vi "open.vi"(8 "error in (no error)":errorcluster caption="错误输入（无错误）", 11 "TCP 输入":refnum<class "TCP.lvclass">) -> (0 "error out":errorcluster caption="错误输出", 3 "TCP 输出":refnum<class "TCP.lvclass">)   [LabVIEW 2016, in "中水三立SQL数据传输.lvlib" / "TCP.lvclass"]
uses:
  TCP.lvclass
  data_inter/data_inter.lvclass/data_inter.ctl
  data_inter/data_inter.lvclass
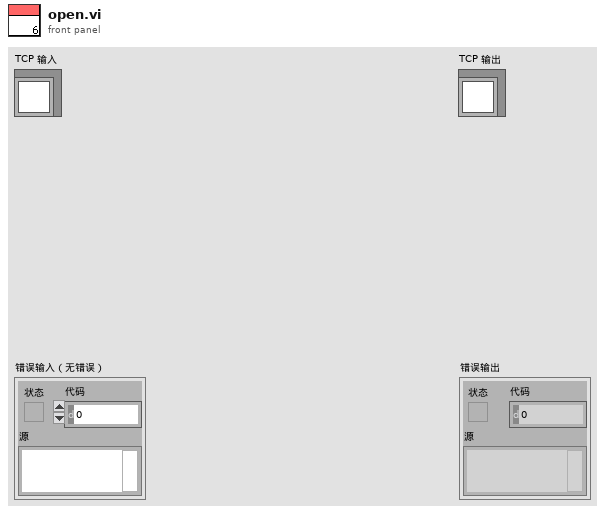
[diagram p1: front panel]
types:
  T1 = cluster{"IP":string, "PORT":string, "VISA resource name":refnum<visa-resource-name>, "baud rate":u32}
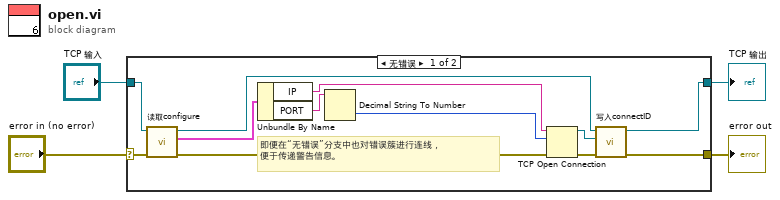
[diagram p0: block diagram]
diagram:
  n1 = case shown="无错误" "error in (no error)" {
    selector: "error in (no error)" -> [w11 w18]
    tunnel: [w6 w18] -> w1
    tunnel: [w5 w17] -> w2
    tunnel: "TCP 输入" -> [w13 w17]
    frame No Error {
      # "即便在“无错误”分支中也对错误簇进行连线，\n便于传递警告信息。"
      n2 = call "读取configure.vi"("error in (no error)"=w11, "data_inter输入"=w13) -> ("error out"=w8:errorcluster, "configure"=w12:T1, "data_inter输出"=w9:refnum<class "TCP.lvclass">)  [unwired: 7 in]
      n3 = Unbundle By Name(w12) -> ("IP"=w14:string, "PORT"=w15:string)
      n4 = Decimal String To Number(string=w15) -> (number=w16:i32)  [unwired: 2 in, 1 out]
      n5 = TCP Open Connection(address=w14, remote port or service name=w16, error in (no error)=w8) -> (connection ID=w10:refnum<k5>, error out=w7:errorcluster)  [unwired: 2 in]
      n6 = call-dynamic "写入connectID.vi"("error in (no error)"=w7, "connectID"=w10, "data_inter输入"=w9) -> ("error out"=w6:errorcluster, "data_inter输出"=w5:refnum<class "TCP.lvclass">)  [unwired: 7 in]
    }
    frame Error {
    }
  }
  "error out" <- w1
  "TCP 输出" <- w2
